vi "TruncCXT.vi"(5 "Decimal places":i8, 6 "Number":cxt format="%#.10f") -> (2 "Truncated number":cxt format="%#.10f")   [LabVIEW 2017, in "GPNumeric.lvlib"]
doc: "Truncates both the real and imaginary parts of the complex <B>Number</B> to a number of <B>Decimal places</B>.\n\nYou can set <B>Decimal places</B> to a negative number to truncate to nearest 10, nearest 100 and so on. E.g. to truncate 782-55i to the nearest hundred, you set <B>Decimal places</B> to -2 and the <B>Truncated number</B> will be 700-0i.\n\nThis VI is inlined.\n\nSteen Schmidt\nGPower\n6/4 2014"
uses:
  GPNumeric.lvlib
panel:
  # "Copyright © 2014\nGPower\nSee enclosed license file for terms and conditions"
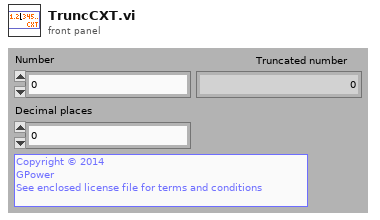
[diagram p1: front panel]
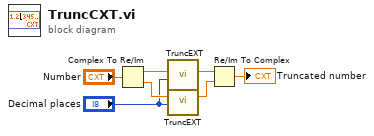
[diagram p0: block diagram]
diagram:
  n1 = Complex To Re/Im(x + iy="Number") -> (x=w7:ext, y=w6:ext)
  n2 = call "TruncEXT.vi"("Decimal places"="Decimal places", "Number"=w7) -> ("Truncated number"=w5:ext)  [unwired: 5 in]
  n3 = call "TruncEXT.vi"("Decimal places"="Decimal places", "Number"=w6) -> ("Truncated number"=w4:ext)  [unwired: 5 in]
  n4 = Re/Im To Complex(1:w4, 2:w5) -> (0:→"Truncated number":cxt)
